vi "Exchange Subsequences.vi"(9 "Subsequence 2":i32[](array[numeric]), 10 "Subsequence 1":u16[](array[numeric]), 11 "Schedule In":u16[](array[numeric])) -> (3 "Child Out":u16[](array[numeric]))   [LabVIEW 2013, in "GA.lvclass"]
uses:
  GA.lvclass
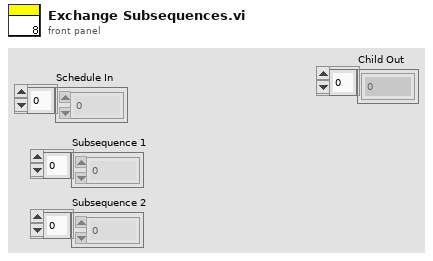
[diagram p1: front panel]
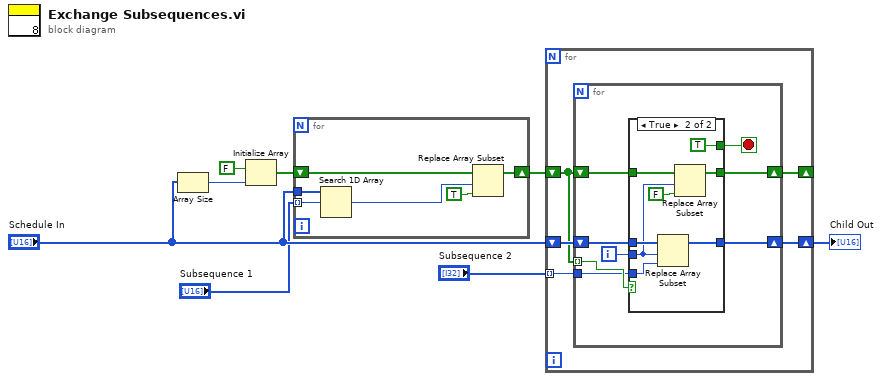
[diagram p0: block diagram]
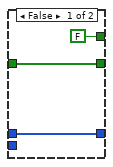
[diagram p2: hidden frame]
diagram:
  n1 = Array Size(array="Schedule In") -> (size(s)=w4:i32)
  n2 = Initialize Array(FALSE, w4) -> (w6:bool[])
  n3 = for {
    tunnel: "Schedule In" -> [w14]
    tunnel: "Subsequence 1" -> [w10] mode=indexing
    shift-right: [w9] -> w3
    shift-left: w6 -> [w13]
    n4 = Search 1D Array(1D array=w14, element=w10) -> (index of element=w11:i32)  [unwired: 1 in]
    n5 = Replace Array Subset(array=w13, new element=TRUE ("new element/subarray"), index=w11) -> (w9:bool[])
  }
  n6 = for {
    tunnel: "Subsequence 2" -> [w19] mode=indexing
    shift-right: [w17] -> w8
    shift-left: "Schedule In" -> [w18]
    shift-right: [w15] -> _
    shift-left: w3 -> [w16]
    n7 = for {
      tunnel: w16 -> [w27] mode=indexing
      tunnel: w19 -> [w24]
      shift-right: [w25] -> w17
      shift-left: w18 -> [w26]
      shift-right: [w21] -> w15
      shift-left: w16 -> [w22]
      i -> [w23]
      stop <- w20 stop-if-true
      n8 = case shown="True" w27 {
        tunnel: w26 -> [w30 w38]
        tunnel: [w30 w36] -> w25
        tunnel: w24 -> [_ w37]
        tunnel: w23 -> [_ w34]
        tunnel: w22 -> [w29 w35]
        tunnel: [w29 w32] -> w21
        tunnel: [FALSE TRUE] -> w20
        frame False {
        }
        frame True {
          n9 = Replace Array Subset(array=w38, new element=w37, index=w34) -> (w36:u16[])
          n10 = Replace Array Subset(array=w35, new element=FALSE ("new element/subarray"), index=w34) -> (w32:bool[])
        }
      }
    }
  }
  "Child Out" <- w8
